vi "Begin.vi"(11 "Image Size":T1=enum."160x120") -> (0 "error out":errorcluster)   [LabVIEW 2012]
doc: "Called before other user functions, this VI is expected to open initial I/O refnums, load in file data, and do all program initialization. Notice that the <B>error out</B> terminal is simply used for data flow. Wiring it to other structures or subVIs ensures that this VI runs first."
uses:
  <vilib>/Rock Robotics/WPI/Camera/WPI_CameraImageSize.ctl
  <vilib>/Rock Robotics/WPI/DriverStation/WPI_DriverStationRobotMode2.ctl
  <vilib>/Rock Robotics/SystemInterfaces/Typedef/FPGA_TypedefDigitalModule.ctl
  <vilib>/Rock Robotics/SystemInterfaces/DIO/FPGA_DIOPWMChannel.ctl
  <vilib>/Rock Robotics/SystemInterfaces/DIO/FPGA_DIOChannel.ctl
  <vilib>/Rock Robotics/SystemInterfaces/DIO/FPGA_DIORelayChannel.ctl
  <vilib>/Rock Robotics/WPI/Relay/WPI_RelayDirection.ctl
  <vilib>/Rock Robotics/WPI/Encoder/WPI_EncoderType.ctl
  <vilib>/Rock Robotics/WPI/Joystick/WPI_JoystickDeviceEnum.ctl
  <vilib>/Rock Robotics/SystemInterfaces/Typedef/FPGA_TypedefAnalogModule.ctl
  <vilib>/Rock Robotics/SystemInterfaces/AI/FPGA_AIChannel.ctl
  <vilib>/Rock Robotics/WPI/SafetyOutput/WPI_SafetyOutputConfigMenu.ctl
  Extra Project/2013 Robot Motors/Robot Global Data.vi
  <vilib>/Rock Robotics/WPI/MotorControl/WPI_MotorControlOpen Victor.vi
  <vilib>/Rock Robotics/WPI/MotorControl/WPI_MotorControlOpen Jaguar.vi
  <vilib>/Rock Robotics/WPI/Counter/WPI_CounterDigitalInputToDigitalSource.vi
  <vilib>/Rock Robotics/WPI/RobotDrive/WPI_RobotDriveOpen2MotorWithJaguar.vi
  <vilib>/Rock Robotics/WPI/Camera/WPI_CameraWhite Balance Values.ctl
  <vilib>/Rock Robotics/WPI/Camera/WPI_CameraExposure Values.ctl
  <vilib>/Rock Robotics/WPI/Camera/WPI_CameraFrameRate.ctl
  <vilib>/Rock Robotics/WPI/RobotDrive/WPI_RobotDriveOpen4MotorWithJaguar.vi
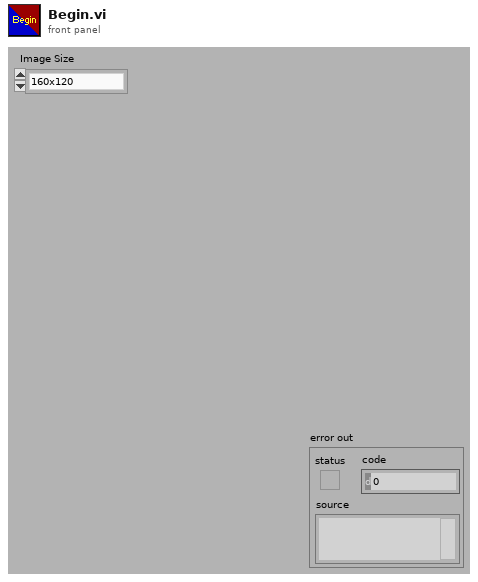
[diagram p1: front panel]
types:
  T1 = typedef "WPI_CameraImageSize.ctl" = enum16{"640x480", "320x240", "160x120"}
  T2 = typedef "WPI_DriverStationRobotMode2.ctl" = enum16{"Autonomous Disabled", "Autonomous Enabled", "Teleop Disabled", "Teleop Enabled", "Timeout", "Finish", "Test Disabled", "Test Enabled"}
  T3 = typedef "WPI_CameraFrameRate.ctl" = u32
  T4 = typedef "WPI_CameraExposure Values.ctl" = enum16{"Auto", "Flicker-free 50 Hz", "Flicker-free 60 Hz", "Hold current"}
  T5 = typedef "WPI_CameraWhite Balance Values.ctl" = enum16{"Auto", "Fixed indoor", "Fixed outdoor 1", "Fixed outdoor 2", "Fixed fluorescent 1", "Fixed fluorescent 2", "Hold current"}
  T6 = typedef "WPI_CameraDevRef.ctl" = cluster{"Camera Address":string, "CameraStatus":errorcluster, "Acquire Image Notifier":refnum<notifier>}
  T7 = typedef "FPGA_DIOChannel.ctl" = enum8{"DIO 1", "DIO 2", "DIO 3", "DIO 4", "DIO 5", "DIO 6", "DIO 7", "DIO 8", "DIO 9", "DIO 10", "DIO 11", "DIO 12", "DIO 13", "DIO 14", "Invalid"}
  T8 = typedef "FPGA_TypedefDigitalModule.ctl" = enum16{"Digital Module 1", "Digital Module 2"}
  T9 = typedef "WPI_DigitalInputDevRef.ctl" = cluster{"DevStatus":errorcluster, "DIO Channel":T7, "Digital Module":T8}
  T10 = typedef "WPI_SafetyOutputConfigMenu.ctl" = enum16{"Enable", "Disable"}
  T11 = typedef "FPGA_DIOPWMChannel.ctl" = enum8{"PWM 1", "PWM 2", "PWM 3", "PWM 4", "PWM 5", "PWM 6", "PWM 7", "PWM 8", "PWM 9", "PWM 10", "Invalid"}
  T12 = typedef "WPI_RobotDriveDevRef.ctl" = cluster{"DevStatus":errorcluster, "Motors[]":T13[], "Square Inputs":bool, "Max Output":dbl, "Isochronous":bool}
  T13 = typedef "WPI_MotorControlDeviceRef.ctl" = cluster{"DeviceStatus":errorcluster, "Type":enum16{"PWM", "CAN"}, "PWM":cluster{"Digital Module":T8, "PWM Channel":T11, "DeadBand":T14}, "CAN":cluster{"Device Number":u8, "Control Mode":T15, "Semaphore":T16, "Max Vout":dbl}, "Invert":bool, "TransformRef":T17, "InvTransformRef":T17}
  T14 = typedef "WPI_PWMDeadband.ctl" = cluster{"Name":string, "maxPositivePwm":i32, "minPositivePwm":i32, "centerPwm":i32, "maxNegativePwm":i32, "minNegativePwm":i32, "angularRange":u16}
  T15 = typedef "WPI_CANJaguar_ControlMode.ctl" = enum8{"Percent VBus", "Current", "Speed", "Position", "Voltage"}
  T16 = typedef "Semaphore RefNum" = refnum<k1>
  T17 = typedef "WPI_PWMTransform_ConPane.ctl" = refnum<vi>
  T18 = typedef "WPI_RelayDirection.ctl" = enum16{"Both directions", "Forward only", "Reverse only"}
  T19 = typedef "FPGA_DIORelayChannel.ctl" = enum8{"Relay 1", "Relay 2", "Relay 3", "Relay 4", "Relay 5", "Relay 6", "Relay 7", "Relay 8", "Invalid"}
  T20 = typedef "WPI_ServoDeviceRef.ctl" = cluster{"DeviceStatus":errorcluster, "Digital Module":T8, "PWM Channel":T11, "DeadBand":T14}
  T21 = typedef "WPI_RelayDevRef.ctl" = cluster{"DevStatus":errorcluster, "Relay Channel":T19, "Digital Module":T8, "Relay Direction":T18}
  T22 = typedef "WPI_JoystickDeviceEnum.ctl" = enum16{"USB 1", "USB 2", "USB 3", "USB 4", "Kinect 1", "Kinect 2"}
  T23 = typedef "WPI_JoystickDevRef.ctl" = cluster{"Device":T22}
  T24 = typedef "WPI_EncoderType.ctl" = enum16{"1x", "2x", "4x"}
  T25 = typedef "FPGA_CounterEncoderSourceConvertionLVSourceType.ctl" = cluster{"DevStatus":errorcluster, "AnalogTriggerMode?":bool, "DigitalMode":cluster{"Digital Module":T8, "DIO Channel":T26}, "AnalogTriggerMode":cluster{"AnalogTriggerIndex":T27, "OutputType":T28}}
  T26 = typedef "FPGA_DIODigitalSourceChannel.ctl" = enum8{"DIO 1", "DIO 2", "DIO 3", "DIO 4", "DIO 5", "DIO 6", "DIO 7", "DIO 8", "DIO 9", "DIO 10", "DIO 11", "DIO 12", "DIO 13", "DIO 14", "Disabled"}
  T27 = typedef "FPGA_AnalogTriggerIndex.ctl" = enum8{"Trig 0", "Trig 1", "Trig 2", "Trig 3", "Trig 4", "Trig 5", "Trig 6", "Trig 7", "Invalid"}
  T28 = typedef "FPGA_AnalogTriggerOutType.ctl" = enum16{"InWindow", "TriggerState", "Rising", "Falling"}
  T29 = typedef "WPI_EncoderDevRef.ctl" = cluster{"DevStatus":errorcluster, "EncoderIndex":T30, "CounterIndex":T31, "DistancePerCount":dbl, "Decoding Type":T24}
  T30 = typedef "FPGA_EncoderIdx.ctl" = enum8{"Enc 0", "Enc 1", "Enc 2", "Enc 3", "Invalid"}
  T31 = typedef "FPGA_CounterCtrSystemIndex.ctl" = enum8{"Ctr 0", "Ctr 1", "Ctr 2", "Ctr 3", "Ctr 4", "Ctr 5", "Ctr 6", "Ctr 7", "Invalid"}
  T32 = typedef "FPGA_AIChannel.ctl" = enum8{"AI 1", "AI 2", "AI 3", "AI 4", "AI 5", "AI 6", "AI 7", "AI 8", "Invalid"}
  T33 = typedef "FPGA_TypedefAnalogModule.ctl" = enum16{"Analog Module 1", "Analog Module 2"}
  T34 = typedef "WPI_AnalogChannelDevRef.ctl" = cluster{"DevStatus":errorcluster, "Analog Module":T33, "Analog Channel":T32}
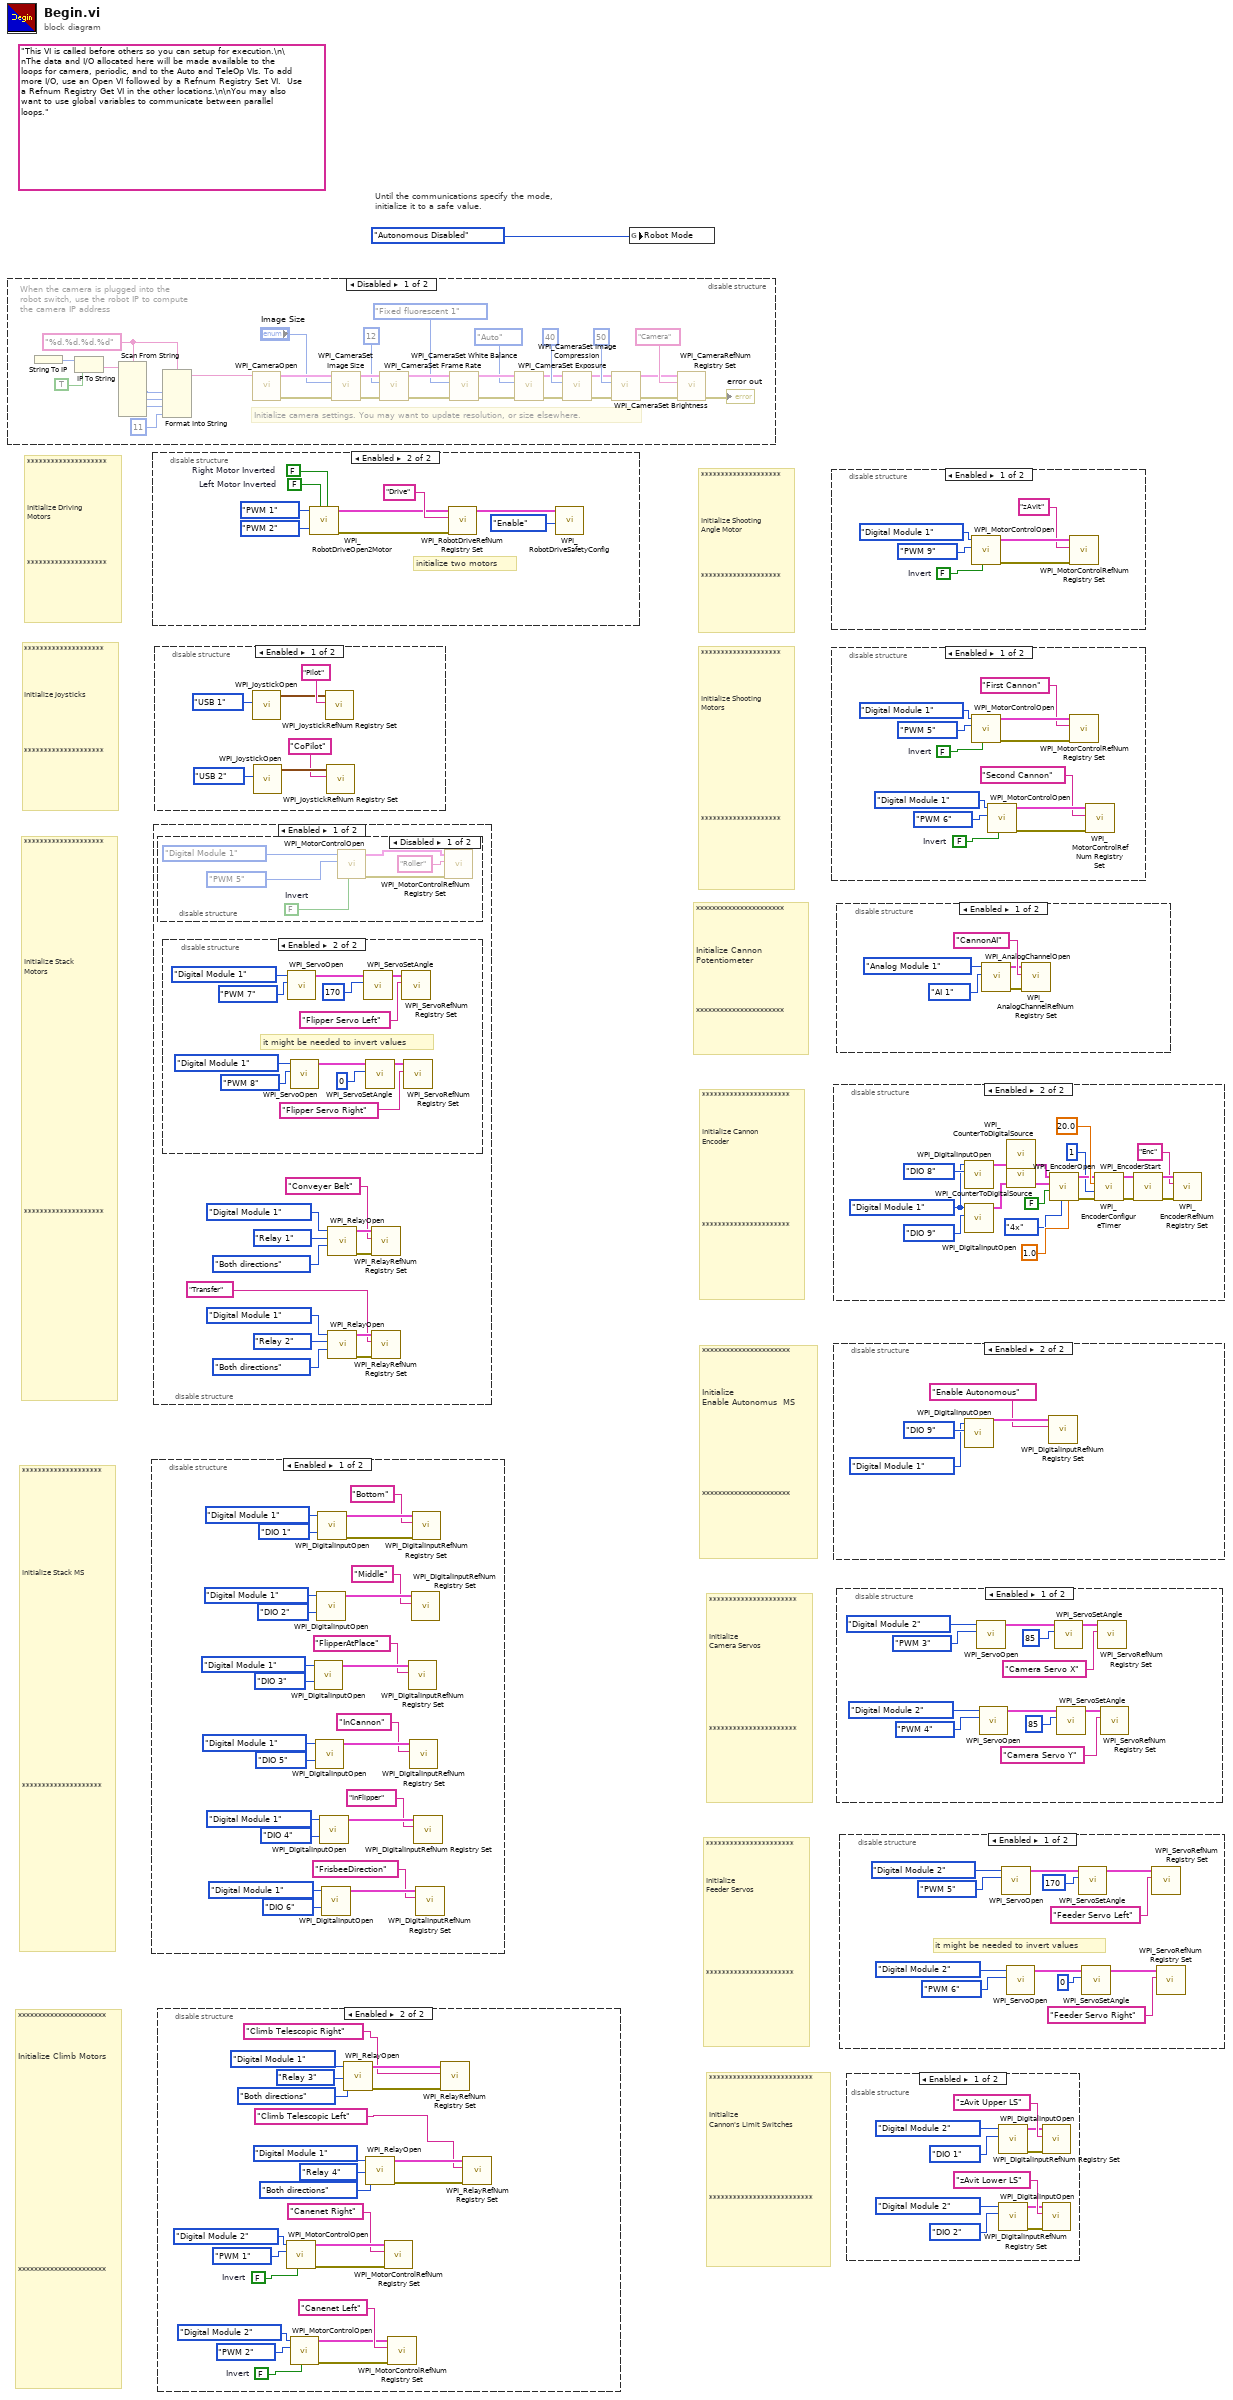
[diagram p0: block diagram]
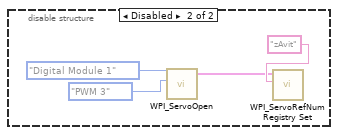
[diagram p7: hidden frame]
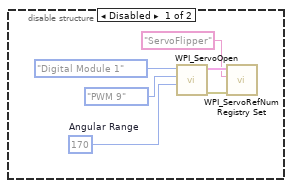
[diagram p14: hidden frame]
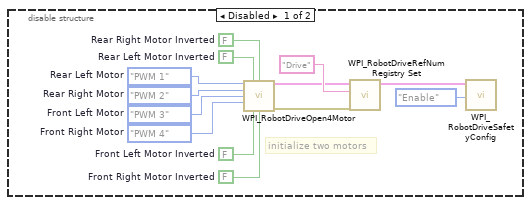
[diagram p16: hidden frame]
diagram:
  (unwired) "This VI is called before others so you can setup for execution.\n\nThe data and I/O allocated here will be made available to the loops for camera, periodic, and to the Auto and TeleOp VIs. To add more I/O, use an Open VI followed by a Refnum Registry Set VI.  Use a Refnum Registry Get VI in the other locations.\n\nYou may also want to use global variables to communicate between parallel loops."
  # "**************************\n\n\n\nInitialize\nCannon's Limit Switches\n\n\n\n\n\n\n\n**************************"
  # "**********************\n\n\n\nInitialize\nFeeder Servos\n\n\n\n\n\n\n\n\n**********************"
  # "**********************\n\n\n\nInitialize\nCamera Servos\n\n\n\n\n\n\n\n\n**********************"
  # "**********************\n\n\n\nInitialize Climb Motors          \n\n\n\n\n\n\n\n\n\n\n\n\n\n\n\n\n\n\n\n\n**********************"
  # "**********************\n\n\n\nInitialize\nEnable Autonomus  MS\n\n\n\n\n\n\n\n\n**********************"
  # "********************\n\n\n\n\nInitialize Shooting\nAngle Motor\n\n\n\n\n********************"
  # "**********************\n\n\n           \nInitialize Cannon Potentiometer\n\n\n\n\n**********************"
  # "**********************\n\n\n\nInitialize Cannon\nEncoder           \n\n\n\n\n\n\n\n\n**********************"
  # "********************\n\n\n\n\n\n\n\n\n\n\nInitialize Stack MS\n\n\n\n\n\n\n\n\n\n\n\n\n\n\n\n\n\n\n\n\n\n\n********************"
  # "********************\n\n\n\n\nInitialize Shooting\nMotors\n\n\n\n\n\n\n\n\n\n\n\n********************"
  # "********************\n\n\n\n\n\n\n\n\n\n\n\n\nInitialize Stack \nMotors\n\n\n\n\n\n\n\n\n\n\n\n\n\n\n\n\n\n\n\n\n\n\n\n\n\n********************"
  # "********************\n\n\n\n\nInitialize Driving\nMotors\n\n\n\n\n********************"
  # "********************\n\n\n\n\nInitialize Joysticks\n\n\n\n\n\n********************"
  # "Until the communications specify the mode,\ninitialize it to a safe value."
  n1 = disable-structure shown="Disabled" {
    frame Disabled {
      w4 = "%d.%d.%d.%d" ("format string")
      # "When the camera is plugged into the\nrobot switch, use the robot IP to compute\nthe camera IP address"
      # "Initialize camera settings. You may want to update resolution, or size elsewhere."
      n2 = String To IP() -> (0:w11:u32)  [unwired: 1 in]
      n3 = IP To String(1:TRUE ("dot notation? (F)"), 2:w11) -> (0:w9:string)
      n4 = Scan From String(format string=w4, input string=w9) -> (output 1=w8:i32, output 2=w7:i32, output 3=w6:i32)  [unwired: 7 in, 3 out]
      n5 = Format Into String(format string=w4, w8, w7, w6, 11 ("Compression")) -> (resulting string=w3:string)  [unwired: 2 in, 1 out]
      n6 = call <vilib>:"WPI_CameraOpen.vi"("Camera Address"=w3) -> ("error out"=w23:errorcluster, "CameraDevRef"=w24:T6)  [unwired: 2 in, 7 out]
      n7 = call <vilib>:"WPI_CameraSet Image Size.vi"("error in (no error)"=w23, "Image Size"="Image Size", "CameraDevRef"=w24) -> ("error out"=w22:errorcluster, "CameraDevRef Out"=w25:T6)  [unwired: 7 out]
      n8 = call <vilib>:"WPI_CameraSet Frame Rate.vi"("error in (no error)"=w22, "Frame Rate (fps)"=T3 12, "CameraDevRef"=w25) -> ("error out"=w21:errorcluster, "CameraDevRef Out"=w27:T6)  [unwired: 7 out]
      n9 = call <vilib>:"WPI_CameraSet White Balance.vi"("error in (no error)"=w21, "White Balance"=WPI_CameraWhite_Balance_Values."Fixed fluorescent 1", "CameraDevRef"=w27) -> ("error out"=w20:errorcluster, "CameraDevRef Out"=w26:T6)  [unwired: 7 out]
      n10 = call <vilib>:"WPI_CameraSet Exposure.vi"("error in (no error)"=w20, "Exposure"=WPI_CameraExposure_Values."Auto", "CameraDevRef"=w26) -> ("error out"=w19:errorcluster, "CameraDevRef Out"=w29:T6)  [unwired: 7 out]
      n11 = call <vilib>:"WPI_CameraSet Image Compression.vi"("error in (no error)"=w19, "Compression"=40, "CameraDevRef"=w29) -> ("error out"=w18:errorcluster, "CameraDevRef Out"=w28:T6)  [unwired: 7 out]
      n12 = call <vilib>:"WPI_CameraSet Brightness.vi"("error in (no error)"=w18, "Brightness"=50, "CameraDevRef"=w28) -> ("error out"=w16:errorcluster, "CameraDevRef Out"=w17:T6)  [unwired: 7 out]
      n13 = call <vilib>:"WPI_CameraRefNum Registry Set.vi"("error in (no error)"=w16, "refnum name"="Camera", "CameraDevRef"=w17) -> ("error out"=→"error out":errorcluster)  [unwired: 8 out]
    }
    frame Enabled {
    }
  }
  n14 = disable-structure shown="Enabled" {
    frame Enabled {
      n15 = call <vilib>:"WPI_DigitalInputOpen.vi"("DIO Channel"=FPGA_DIOChannel."DIO 3", "Digital Module (Module 1)"=FPGA_TypedefDigitalModule."Digital Module 1") -> ("DigitalInputDevRef"=w36:T9)  [unwired: 8 in, 1 out]
      n16 = call <vilib>:"WPI_DigitalInputOpen.vi"("DIO Channel"=FPGA_DIOChannel."DIO 5", "Digital Module (Module 1)"=FPGA_TypedefDigitalModule."Digital Module 1") -> ("DigitalInputDevRef"=w50:T9)  [unwired: 8 in, 1 out]
      n17 = call <vilib>:"WPI_DigitalInputOpen.vi"("DIO Channel"=FPGA_DIOChannel."DIO 2", "Digital Module (Module 1)"=FPGA_TypedefDigitalModule."Digital Module 1") -> ("DigitalInputDevRef"=w53:T9)  [unwired: 8 in, 1 out]
      n18 = call <vilib>:"WPI_DigitalInputOpen.vi"("DIO Channel"=FPGA_DIOChannel."DIO 1", "Digital Module (Module 1)"=FPGA_TypedefDigitalModule."Digital Module 1") -> ("error out"=w56:errorcluster, "DigitalInputDevRef"=w57:T9)  [unwired: 8 in]
      n19 = call <vilib>:"WPI_DigitalInputOpen.vi"("DIO Channel"=FPGA_DIOChannel."DIO 4", "Digital Module (Module 1)"=FPGA_TypedefDigitalModule."Digital Module 1") -> ("DigitalInputDevRef"=w47:T9)  [unwired: 8 in, 1 out]
      n20 = call <vilib>:"WPI_DigitalInputOpen.vi"("DIO Channel"=FPGA_DIOChannel."DIO 6", "Digital Module (Module 1)"=FPGA_TypedefDigitalModule."Digital Module 1") -> ("DigitalInputDevRef"=w42:T9)  [unwired: 8 in, 1 out]
      n21 = call <vilib>:"WPI_DigitalInputRefNum Registry Set.vi"("refnum name"="FlipperAtPlace", "DigitalInputDevRef"=w36) -> ()  [unwired: 8 in, 2 out]
      n22 = call <vilib>:"WPI_DigitalInputRefNum Registry Set.vi"("refnum name"="InCannon", "DigitalInputDevRef"=w50) -> ()  [unwired: 8 in, 2 out]
      n23 = call <vilib>:"WPI_DigitalInputRefNum Registry Set.vi"("refnum name"="Middle", "DigitalInputDevRef"=w53) -> ()  [unwired: 8 in, 2 out]
      n24 = call <vilib>:"WPI_DigitalInputRefNum Registry Set.vi"("error in (no error)"=w56, "refnum name"="Bottom", "DigitalInputDevRef"=w57) -> ()  [unwired: 7 in, 2 out]
      n25 = call <vilib>:"WPI_DigitalInputRefNum Registry Set.vi"("refnum name"="InFlipper", "DigitalInputDevRef"=w47) -> ()  [unwired: 8 in, 2 out]
      n26 = call <vilib>:"WPI_DigitalInputRefNum Registry Set.vi"("refnum name"="FrisbeeDirection", "DigitalInputDevRef"=w42) -> ()  [unwired: 8 in, 2 out]
    }
    frame Disabled {
    }
  }
  n27 = disable-structure shown="Enabled" {
    frame Disabled {
      w58 = FPGA_DIOPWMChannel."PWM 4"  # Front Right Motor
      w59 = FPGA_DIOPWMChannel."PWM 3"  # Front Left Motor
      w60 = FPGA_DIOPWMChannel."PWM 2"  # Rear Right Motor
      w61 = FPGA_DIOPWMChannel."PWM 1"  # Rear Left Motor
      w62 = FALSE  # Front Right Motor Inverted
      w63 = FALSE  # Front Left Motor Inverted
      w64 = FALSE  # Rear Right Motor Inverted
      w65 = FALSE  # Rear Left Motor Inverted
      # "initialize two motors"
      n28 = call-poly <vilib>:"WPI_RobotDriveOpen4Motor.vi"("Rear Left Motor"=w61, "Rear Left Motor Inverted"=w65, "Rear Right Motor Inverted"=w64, "Rear Right Motor"=w60, "Front Left Motor"=w59, "Front Right Motor"=w58, "Front Left Motor Inverted"=w63, "Front Right Motor Inverted"=w62) -> ("RobotDriveDevRef"=w67:T12, "error out"=w66:errorcluster)  [unwired: 6 in]
      n29 = call <vilib>:"WPI_RobotDriveRefNum Registry Set.vi"("error in (no error)"=w66, "refnum name"="Drive", "RobotDriveDevRef"=w67) -> ("RobotDriveDevRef"=w69:T12)  [unwired: 8 out]
      n30 = call <vilib>:"WPI_RobotDriveSafetyConfig.vi"("mode"=WPI_SafetyOutputConfigMenu."Enable", "RobotDriveDevRef"=w69) -> ()  [unwired: 8 in, 2 out]
    }
    frame Enabled {
      w71 = FALSE  # Right Motor Inverted
      w72 = FALSE  # Left Motor Inverted
      # "initialize two motors"
      n31 = call-poly <vilib>:"WPI_RobotDriveOpen2Motor.vi"("Right Motor Inverted"=w71, "Left Motor Inverted"=w72, "Right Motor"=FPGA_DIOPWMChannel."PWM 2", "Left Motor"=FPGA_DIOPWMChannel."PWM 1") -> ("error out"=w75:errorcluster, "RobotDriveDevRef"=w76:T12)  [unwired: 6 in]
      n32 = call <vilib>:"WPI_RobotDriveRefNum Registry Set.vi"("error in (no error)"=w75, "refnum name"="Drive", "RobotDriveDevRef"=w76) -> ("RobotDriveDevRef"=w78:T12)  [unwired: 8 out]
      n33 = call <vilib>:"WPI_RobotDriveSafetyConfig.vi"("mode"=WPI_SafetyOutputConfigMenu."Enable", "RobotDriveDevRef"=w78) -> ()  [unwired: 8 in, 2 out]
    }
  }
  n34 = disable-structure shown="Enabled" {
    frame Enabled {
      n35 = disable-structure shown="Disabled" {
        frame Disabled {
          w93 = FALSE  # Invert
          n36 = call-poly <vilib>:"WPI_MotorControlOpen.vi"("Invert"=w93, "PWM Channel"=FPGA_DIOPWMChannel."PWM 5", "Digital Module (Module 1)"=FPGA_TypedefDigitalModule."Digital Module 1") -> ("error out"=w92:errorcluster, "MotorControlDeviceRef"=w97:T13)  [unwired: 7 in]
          n37 = call <vilib>:"WPI_MotorControlRefNum Registry Set.vi"("error in (no error)"=w92, "refnum name"="Roller", "MotorControlDevRef"=w97) -> ()  [unwired: 7 in, 2 out]
        }
        frame Enabled {
        }
      }
      n38 = disable-structure shown="Enabled" {
        frame Disabled {
          w100 = u16 170  # Angular Range
          n39 = call <vilib>:"WPI_ServoOpen.vi"("Angular Range"=w100, "PWM Channel"=FPGA_DIOPWMChannel."PWM 9", "Digital Module (Module 1)"=FPGA_TypedefDigitalModule."Digital Module 1") -> ("error out"=w99:errorcluster, "ServoDeviceRef"=w103:T20)  [unwired: 7 in]
          n40 = call <vilib>:"WPI_ServoRefNum Registry Set.vi"("error in (no error)"=w99, "refnum name"="ServoFlipper", "ServoDeviceRef"=w103) -> ()  [unwired: 7 in, 2 out]
        }
        frame Enabled {
          # "it might be needed to invert values"
          n41 = call <vilib>:"WPI_ServoOpen.vi"("PWM Channel"=FPGA_DIOPWMChannel."PWM 7", "Digital Module (Module 1)"=FPGA_TypedefDigitalModule."Digital Module 1") -> ("ServoDeviceRef"=w115:T20)  [unwired: 8 in, 1 out]
          n42 = call <vilib>:"WPI_ServoOpen.vi"("PWM Channel"=FPGA_DIOPWMChannel."PWM 8", "Digital Module (Module 1)"=FPGA_TypedefDigitalModule."Digital Module 1") -> ("ServoDeviceRef"=w105:T20)  [unwired: 8 in, 1 out]
          n43 = call <vilib>:"WPI_ServoSetAngle.vi"("Angle"=170, "ServoDeviceRef"=w115) -> ("ServoDeviceRef"=w111:T20)  [unwired: 8 in, 1 out]
          n44 = call <vilib>:"WPI_ServoSetAngle.vi"("Angle"=0, "ServoDeviceRef"=w105) -> ("ServoDeviceRef"=w108:T20)  [unwired: 8 in, 1 out]
          n45 = call <vilib>:"WPI_ServoRefNum Registry Set.vi"("refnum name"="Flipper Servo Left", "ServoDeviceRef"=w111) -> ()  [unwired: 8 in, 2 out]
          n46 = call <vilib>:"WPI_ServoRefNum Registry Set.vi"("refnum name"="Flipper Servo Right", "ServoDeviceRef"=w108) -> ()  [unwired: 8 in, 2 out]
        }
      }
      n47 = call <vilib>:"WPI_RelayOpen.vi"("Relay Direction"=WPI_RelayDirection."Both directions", "Relay Channel"=FPGA_DIORelayChannel."Relay 1", "Digital Module (Module 1)"=FPGA_TypedefDigitalModule."Digital Module 1") -> ("error out"=w90:errorcluster, "RelayDevRef"=w91:T21)  [unwired: 7 in]
      n48 = call <vilib>:"WPI_RelayOpen.vi"("Relay Direction"=WPI_RelayDirection."Both directions", "Relay Channel"=FPGA_DIORelayChannel."Relay 2", "Digital Module (Module 1)"=FPGA_TypedefDigitalModule."Digital Module 1") -> ("error out"=w83:errorcluster, "RelayDevRef"=w82:T21)  [unwired: 7 in]
      n49 = call <vilib>:"WPI_RelayRefNum Registry Set.vi"("error in (no error)"=w90, "refnum name"="Conveyer Belt", "RelayDevRef"=w91) -> ()  [unwired: 7 in, 2 out]
      n50 = call <vilib>:"WPI_RelayRefNum Registry Set.vi"("error in (no error)"=w83, "refnum name"="Transfer", "RelayDevRef"=w82) -> ()  [unwired: 7 in, 2 out]
    }
    frame Disabled {
    }
  }
  n51 = disable-structure shown="Enabled" {
    frame Enabled {
      n52 = call <vilib>:"WPI_JoystickOpen.vi"("JoystickDevice"=WPI_JoystickDeviceEnum."USB 1") -> ("JoystickDevRef"=w120:T23)  [unwired: 10 in]
      n53 = call <vilib>:"WPI_JoystickOpen.vi"("JoystickDevice"=WPI_JoystickDeviceEnum."USB 2") -> ("JoystickDevRef"=w117:T23)  [unwired: 10 in]
      n54 = call <vilib>:"WPI_JoystickRefNum Registry Set.vi"("refnum name"="Pilot", "JoystickDevRef"=w120) -> ()  [unwired: 8 in, 2 out]
      n55 = call <vilib>:"WPI_JoystickRefNum Registry Set.vi"("refnum name"="CoPilot", "JoystickDevRef"=w117) -> ()  [unwired: 8 in, 2 out]
    }
    frame Disabled {
    }
  }
  n56 = disable-structure shown="Enabled" {
    frame Disabled {
    }
    frame Enabled {
      w138 = FALSE  # Invert
      w141 = FALSE  # Invert
      n57 = call-poly <vilib>:"WPI_MotorControlOpen.vi"("Invert"=w141, "PWM Channel"=FPGA_DIOPWMChannel."PWM 1", "Digital Module (Module 1)"=FPGA_TypedefDigitalModule."Digital Module 2") -> ("error out"=w140:errorcluster, "MotorControlDeviceRef"=w145:T13)  [unwired: 7 in]
      n58 = call-poly <vilib>:"WPI_MotorControlOpen.vi"("Invert"=w138, "PWM Channel"=FPGA_DIOPWMChannel."PWM 2", "Digital Module (Module 1)"=FPGA_TypedefDigitalModule."Digital Module 2") -> ("error out"=w139:errorcluster, "MotorControlDeviceRef"=w134:T13)  [unwired: 7 in]
      n59 = call <vilib>:"WPI_RelayOpen.vi"("Relay Direction"=WPI_RelayDirection."Both directions", "Relay Channel"=FPGA_DIORelayChannel."Relay 3", "Digital Module (Module 1)"=FPGA_TypedefDigitalModule."Digital Module 1") -> ("error out"=w132:errorcluster, "RelayDevRef"=w133:T21)  [unwired: 7 in]
      n60 = call <vilib>:"WPI_RelayOpen.vi"("Relay Direction"=WPI_RelayDirection."Both directions", "Relay Channel"=FPGA_DIORelayChannel."Relay 4", "Digital Module (Module 1)"=FPGA_TypedefDigitalModule."Digital Module 1") -> ("error out"=w126:errorcluster, "RelayDevRef"=w127:T21)  [unwired: 7 in]
      n61 = call <vilib>:"WPI_MotorControlRefNum Registry Set.vi"("error in (no error)"=w140, "refnum name"="Canenet Right", "MotorControlDevRef"=w145) -> ()  [unwired: 7 in, 2 out]
      n62 = call <vilib>:"WPI_MotorControlRefNum Registry Set.vi"("error in (no error)"=w139, "refnum name"="Canenet Left", "MotorControlDevRef"=w134) -> ()  [unwired: 7 in, 2 out]
      n63 = call <vilib>:"WPI_RelayRefNum Registry Set.vi"("error in (no error)"=w132, "refnum name"="Climb Telescopic Right", "RelayDevRef"=w133) -> ()  [unwired: 7 in, 2 out]
      n64 = call <vilib>:"WPI_RelayRefNum Registry Set.vi"("error in (no error)"=w126, "refnum name"="Climb Telescopic Left", "RelayDevRef"=w127) -> ()  [unwired: 7 in, 2 out]
    }
  }
  n65 = global write "Robot Global Data.vi" "Robot Mode"(WPI_DriverStationRobotMode2."Autonomous Disabled" ("Robot Mode")) -> ()
  n66 = disable-structure shown="Enabled" {
    frame Enabled {
      w147 = FALSE  # Invert
      n67 = call-poly <vilib>:"WPI_MotorControlOpen.vi"("Invert"=w147, "PWM Channel"=FPGA_DIOPWMChannel."PWM 9", "Digital Module (Module 1)"=FPGA_TypedefDigitalModule."Digital Module 1") -> ("error out"=w146:errorcluster, "MotorControlDeviceRef"=w151:T13)  [unwired: 7 in]
      n68 = call <vilib>:"WPI_MotorControlRefNum Registry Set.vi"("error in (no error)"=w146, "refnum name"="zAvit", "MotorControlDevRef"=w151) -> ()  [unwired: 7 in, 2 out]
    }
    frame Disabled {
      n69 = call <vilib>:"WPI_ServoOpen.vi"("PWM Channel"=FPGA_DIOPWMChannel."PWM 3", "Digital Module (Module 1)"=FPGA_TypedefDigitalModule."Digital Module 1") -> ("ServoDeviceRef"=w152:T20)  [unwired: 8 in, 1 out]
      n70 = call <vilib>:"WPI_ServoRefNum Registry Set.vi"("refnum name"="zAvit", "ServoDeviceRef"=w152) -> ()  [unwired: 8 in, 2 out]
    }
  }
  n71 = disable-structure shown="Enabled" {
    frame Enabled {
      w157 = FALSE  # Invert
      w163 = FALSE  # Invert
      n72 = call-poly <vilib>:"WPI_MotorControlOpen.vi"("Invert"=w163, "PWM Channel"=FPGA_DIOPWMChannel."PWM 5", "Digital Module (Module 1)"=FPGA_TypedefDigitalModule."Digital Module 1") -> ("error out"=w162:errorcluster, "MotorControlDeviceRef"=w167:T13)  [unwired: 7 in]
      n73 = call-poly <vilib>:"WPI_MotorControlOpen.vi"("Invert"=w157, "PWM Channel"=FPGA_DIOPWMChannel."PWM 6", "Digital Module (Module 1)"=FPGA_TypedefDigitalModule."Digital Module 1") -> ("error out"=w156:errorcluster, "MotorControlDeviceRef"=w161:T13)  [unwired: 7 in]
      n74 = call <vilib>:"WPI_MotorControlRefNum Registry Set.vi"("error in (no error)"=w162, "refnum name"="First Cannon", "MotorControlDevRef"=w167) -> ()  [unwired: 7 in, 2 out]
      n75 = call <vilib>:"WPI_MotorControlRefNum Registry Set.vi"("error in (no error)"=w156, "refnum name"="Second Cannon", "MotorControlDevRef"=w161) -> ()  [unwired: 7 in, 2 out]
    }
    frame Disabled {
    }
  }
  n76 = disable-structure shown="Enabled" {
    frame Disabled {
    }
    frame Enabled {
      w168 = FPGA_TypedefDigitalModule."Digital Module 1" ("DIO Module")
      n77 = call <vilib>:"WPI_DigitalInputOpen.vi"("DIO Channel"=FPGA_DIOChannel."DIO 8" ("A Channel"), "Digital Module (Module 1)"=w168) -> ("DigitalInputDevRef"=w178:T9)  [unwired: 1 in, 8 out]
      n78 = call <vilib>:"WPI_DigitalInputOpen.vi"("DIO Channel"=FPGA_DIOChannel."DIO 9" ("B Channel"), "Digital Module (Module 1)"=w168) -> ("DigitalInputDevRef"=w179:T9)  [unwired: 1 in, 8 out]
      n79 = call-poly <vilib>:"WPI_CounterToDigitalSource.vi"("DigitalInputDevRef"=w178) -> ("Digital Source"=w177:T25)  [unwired: 6 out]
      n80 = call-poly <vilib>:"WPI_CounterToDigitalSource.vi"("DigitalInputDevRef"=w179) -> ("Digital Source"=w180:T25)  [unwired: 6 out]
      n81 = call <vilib>:"WPI_EncoderOpen.vi"("DistancePerCount"=1.0, "Decoding Type"=WPI_EncoderType."4x", "Invert Direction (False)"=FALSE ("Invert Direction"), "BSource"=w180, "ASource"=w177) -> ("error out"=w184:errorcluster, "EncoderDevRef"=w170:T29)  [unwired: 3 in, 2 out]
      n82 = call <vilib>:"WPI_EncoderConfigureTimer.vi"("error in (no error)"=w184, "Number Samples to Average"=u8 1, "Minimum Rate"=20.0, "EncoderDevRef"=w170) -> ("error out"=w185:errorcluster, "EncoderDevRef"=w171:T29)  [unwired: 6 out]
      n83 = call <vilib>:"WPI_EncoderStart.vi"("error in (no error)"=w185, "EncoderDevRef"=w171) -> ("error out"=w186:errorcluster, "EncoderDevRef"=w183:T29)  [unwired: 8 out]
      n84 = call <vilib>:"WPI_EncoderRefNum Registry Set.vi"("error in (no error)"=w186, "refnum name"="Enc", "EncoderDevRef"=w183) -> ()  [unwired: 9 out]
    }
  }
  n85 = disable-structure shown="Enabled" {
    frame Disabled {
    }
    frame Enabled {
      n86 = call <vilib>:"WPI_DigitalInputOpen.vi"("DIO Channel"=FPGA_DIOChannel."DIO 9" ("A Channel"), "Digital Module (Module 1)"=FPGA_TypedefDigitalModule."Digital Module 1" ("DIO Module")) -> ("DigitalInputDevRef"=w188:T9)  [unwired: 1 in, 8 out]
      n87 = call <vilib>:"WPI_DigitalInputRefNum Registry Set.vi"("refnum name"="Enable Autonomous", "DigitalInputDevRef"=w188) -> ()  [unwired: 8 in, 2 out]
    }
  }
  n88 = disable-structure shown="Enabled" {
    frame Enabled {
      n89 = call <vilib>:"WPI_AnalogChannelOpen.vi"("Analog Channel"=FPGA_AIChannel."AI 1", "Analog Module (Module 1)"=FPGA_TypedefAnalogModule."Analog Module 1") -> ("error out"=w192:errorcluster, "AIDeviceRef"=w191:T34)  [unwired: 8 in]
      n90 = call <vilib>:"WPI_AnalogChannelRefNum Registry Set.vi"("error in (no error)"=w192, "refnum name"="CannonAI", "AIDeviceRef"=w191) -> ()  [unwired: 7 in, 2 out]
    }
    frame Disabled {
    }
  }
  n91 = disable-structure shown="Enabled" {
    frame Enabled {
      n92 = call <vilib>:"WPI_ServoOpen.vi"("PWM Channel"=FPGA_DIOPWMChannel."PWM 3", "Digital Module (Module 1)"=FPGA_TypedefDigitalModule."Digital Module 2") -> ("ServoDeviceRef"=w204:T20)  [unwired: 8 in, 1 out]
      n93 = call <vilib>:"WPI_ServoOpen.vi"("PWM Channel"=FPGA_DIOPWMChannel."PWM 4", "Digital Module (Module 1)"=FPGA_TypedefDigitalModule."Digital Module 2") -> ("ServoDeviceRef"=w199:T20)  [unwired: 8 in, 1 out]
      n94 = call <vilib>:"WPI_ServoSetAngle.vi"("Angle"=85, "ServoDeviceRef"=w204) -> ("ServoDeviceRef"=w203:T20)  [unwired: 8 in, 1 out]
      n95 = call <vilib>:"WPI_ServoSetAngle.vi"("Angle"=85, "ServoDeviceRef"=w199) -> ("ServoDeviceRef"=w200:T20)  [unwired: 8 in, 1 out]
      n96 = call <vilib>:"WPI_ServoRefNum Registry Set.vi"("refnum name"="Camera Servo X", "ServoDeviceRef"=w203) -> ()  [unwired: 8 in, 2 out]
      n97 = call <vilib>:"WPI_ServoRefNum Registry Set.vi"("refnum name"="Camera Servo Y", "ServoDeviceRef"=w200) -> ()  [unwired: 8 in, 2 out]
    }
    frame Disabled {
    }
  }
  n98 = disable-structure shown="Enabled" {
    frame Enabled {
      # "it might be needed to invert values"
      n99 = call <vilib>:"WPI_ServoOpen.vi"("PWM Channel"=FPGA_DIOPWMChannel."PWM 5", "Digital Module (Module 1)"=FPGA_TypedefDigitalModule."Digital Module 2") -> ("ServoDeviceRef"=w216:T20)  [unwired: 8 in, 1 out]
      n100 = call <vilib>:"WPI_ServoOpen.vi"("PWM Channel"=FPGA_DIOPWMChannel."PWM 6", "Digital Module (Module 1)"=FPGA_TypedefDigitalModule."Digital Module 2") -> ("ServoDeviceRef"=w215:T20)  [unwired: 8 in, 1 out]
      n101 = call <vilib>:"WPI_ServoSetAngle.vi"("Angle"=170, "ServoDeviceRef"=w216) -> ("ServoDeviceRef"=w211:T20)  [unwired: 8 in, 1 out]
      n102 = call <vilib>:"WPI_ServoSetAngle.vi"("Angle"=0, "ServoDeviceRef"=w215) -> ("ServoDeviceRef"=w210:T20)  [unwired: 8 in, 1 out]
      n103 = call <vilib>:"WPI_ServoRefNum Registry Set.vi"("refnum name"="Feeder Servo Left", "ServoDeviceRef"=w211) -> ()  [unwired: 8 in, 2 out]
      n104 = call <vilib>:"WPI_ServoRefNum Registry Set.vi"("refnum name"="Feeder Servo Right", "ServoDeviceRef"=w210) -> ()  [unwired: 8 in, 2 out]
    }
    frame Disabled {
    }
  }
  n105 = disable-structure shown="Enabled" {
    frame Enabled {
      n106 = call <vilib>:"WPI_DigitalInputOpen.vi"("DIO Channel"=FPGA_DIOChannel."DIO 1", "Digital Module (Module 1)"=FPGA_TypedefDigitalModule."Digital Module 2") -> ("error out"=w225:errorcluster, "DigitalInputDevRef"=w226:T9)  [unwired: 8 in]
      n107 = call <vilib>:"WPI_DigitalInputOpen.vi"("DIO Channel"=FPGA_DIOChannel."DIO 2", "Digital Module (Module 1)"=FPGA_TypedefDigitalModule."Digital Module 2") -> ("error out"=w224:errorcluster, "DigitalInputDevRef"=w227:T9)  [unwired: 8 in]
      n108 = call <vilib>:"WPI_DigitalInputRefNum Registry Set.vi"("error in (no error)"=w225, "refnum name"="zAvit Upper LS", "DigitalInputDevRef"=w226) -> ()  [unwired: 7 in, 2 out]
      n109 = call <vilib>:"WPI_DigitalInputRefNum Registry Set.vi"("error in (no error)"=w224, "refnum name"="zAvit Lower LS", "DigitalInputDevRef"=w227) -> ()  [unwired: 7 in, 2 out]
    }
    frame Disabled {
    }
  }
